vi "Prepare Glue Config Files.vi"(8 "error in":errorcluster, 11 "Project Root":path) -> (0 "error out":errorcluster, 3 "Config Directory":path)   [LabVIEW 2011]
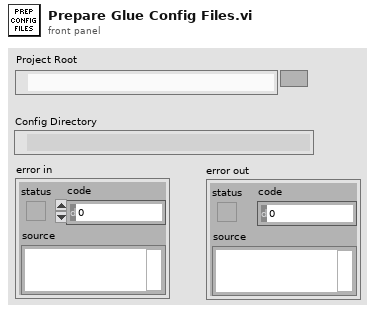
[diagram p1: front panel]
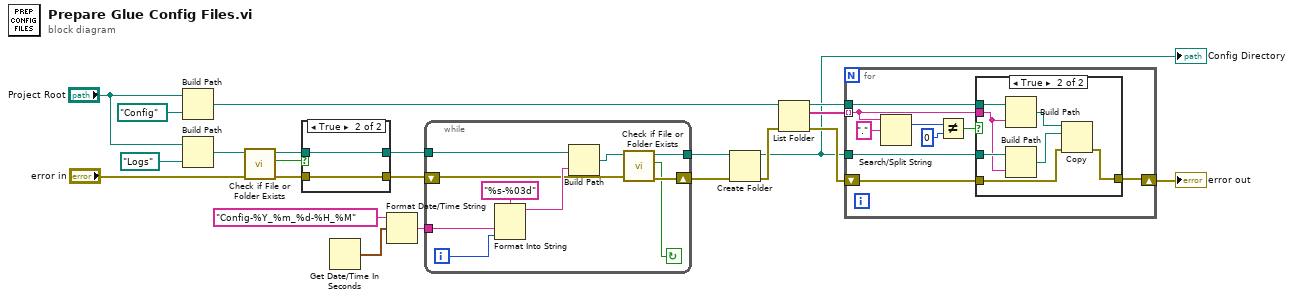
[diagram p0: block diagram]
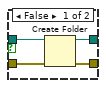
[diagram p3: hidden frame]
diagram:
  n1 = Build Path(base path="Project Root", name or relative path=path "Config") -> (appended path=w6:path)
  n2 = Build Path(base path="Project Root", name or relative path=path "Logs") -> (appended path=w19:path)
  n3 = call <vilib>:"Check if File or Folder Exists.vi"("error in (no error)"="error in", "path"=w19) -> ("error out"=w15:errorcluster, "file or folder exists?"=w17:bool, "dup path"=w16:path)  [unwired: 7 in]
  n4 = case shown="True" w17 {
    tunnel: w16 -> [w26 w28]
    tunnel: w15 -> [w25 w27]
    tunnel: [w24 w28] -> w14
    tunnel: [w23 w27] -> w13
    frame False {
      n5 = Create Folder(path (use dialog)=w26, error in=w25) -> (created path=w24:path, error out=w23:errorcluster)  [unwired: 1 in, 1 out]
    }
    frame True {
    }
  }
  n6 = Get Date/Time In Seconds() -> (seconds since 1Jan1904=w10:timestamp)
  n7 = Format Date/Time String(time format string (%c)="Config-%Y_%m_%d-%H_%M", seconds (now)=w10) -> (date/time string=w12:string)  [unwired: 1 in]
  n8 = while {
    tunnel: w14 -> [w35]
    tunnel: w12 -> [w38]
    shift-right: [w32] -> w8
    shift-left: w13 -> [w33]
    tunnel: [w30] -> w9
    i -> [w37]
    stop <- w31 continue-if-true
    n9 = Format Into String(format string="%s-%03d", w38, w37) -> (resulting string=w36:string)  [unwired: 2 in, 1 out]
    n10 = Build Path(base path=w35, name or relative path=w36) -> (appended path=w34:path)
    n11 = call <vilib>:"Check if File or Folder Exists.vi"("error in (no error)"=w33, "path"=w34) -> ("error out"=w32:errorcluster, "file or folder exists?"=w31:bool, "dup path"=w30:path)  [unwired: 7 in]
  }
  n12 = Create Folder(path (use dialog)=w9, error in=w8) -> (created path=w1:path, error out=w7:errorcluster)  [unwired: 1 in, 1 out]
  "Config Directory" <- w1
  n13 = List Folder(path=w6, error in=w7) -> (path out=w5:path, filenames=w4:string[], error out=w3:errorcluster)  [unwired: 2 in, 1 out]
  n14 = for {
    tunnel: w5 -> [w43]
    tunnel: w4 -> [w42] mode=indexing
    shift-right: [w39] -> w2
    shift-left: w3 -> [w44]
    tunnel: w1 -> [w40]
    n15 = Search/Split String(string=w42, search string/char (-)=".") -> (offset of match=w46:i32)  [unwired: 1 in, 2 out]
    n16 = Not Equal?(x=w46, y=0) -> (x != y?=w41:bool)
    n17 = case shown="True" w41 {
      tunnel: w44 -> [w48 w50]
      tunnel: w43 -> [_ w55]
      tunnel: w42 -> [_ w53]
      tunnel: w40 -> [_ w54]
      tunnel: [w48 w49] -> w39
      frame False {
      }
      frame True {
        n18 = Build Path(base path=w55, name or relative path=w53) -> (appended path=w52:path)
        n19 = Build Path(base path=w54, name or relative path=w53) -> (appended path=w51:path)
        n20 = Copy(8:w50, 10:w51, 11:w52) -> (0:w49:errorcluster)  [unwired: 2 in, 2 out]
      }
    }
  }
  "error out" <- w2
